vi "Array2XYGraphData.vi"(11 "Array in":dbl[][](array[numeric])) -> (3 "Array out":cluster{dbl[], dbl[]}[](array[cluster]))   [LabVIEW 2023]
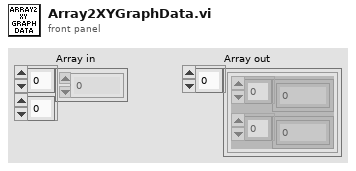
[diagram p1: front panel]
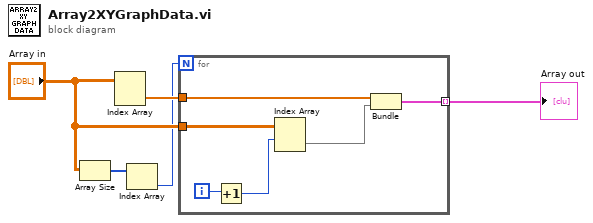
[diagram p0: block diagram]
diagram:
  n1 = Array Size(array="Array in") -> (size(s)=w2:i32[])
  n2 = Index Array(array="Array in") -> (element=w4:dbl[])  [unwired: 2 in]
  n3 = Index Array(array=w2) -> (element=w1:i32)  [unwired: 1 in]
  n4 = for {
    N: w1 -> [_]
    tunnel: w4 -> [w8]
    tunnel: "Array in" -> [w11]
    tunnel: [w6] -> w5 mode=indexing
    i -> [w10]
    n5 = Increment(x=w10) -> (x+1=w9:i32)
    n6 = Index Array(array=w11, index (row)=w9) -> (element=w7:dbl[])  [unwired: 1 in]
    n7 = Bundle("Array in"=w8, "Array in"=w7) -> (w6:cluster{"Array in":dbl[], "Array in":dbl[]})  [unwired: 1 in]
  }
  "Array out" <- w5
